vi "Write lasDiodeData.vi"(8 "error in":errorcluster, 10 "lasDiodeData":waveform(i16), 11 "PAS Cell Data in":refnum<class "PAS Cell Data.lvclass">) -> (0 "error out":errorcluster, 3 "PAS Cell Data out":refnum<class "PAS Cell Data.lvclass">)   [LabVIEW 2018, in "PAS Library.lvlib" / "PAS Cell Data.lvclass"]
doc: "Write the data collected off of the PAS laser diode to the class instance."
uses:
  PAS Cell Data.lvclass
  PAS Cell Data.lvclass/PAS Cell Data.ctl
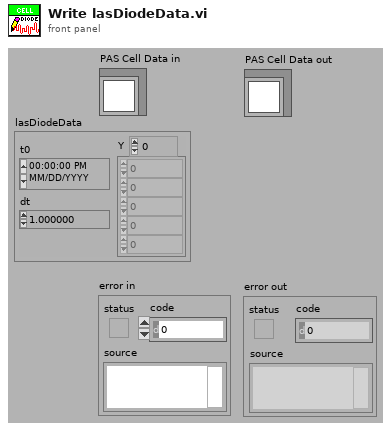
[diagram p1: front panel]
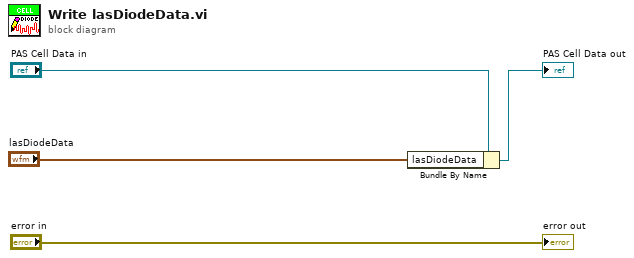
[diagram p0: block diagram]
diagram:
  n1 = Bundle By Name(cluster="PAS Cell Data in", "lasDiodeData"="lasDiodeData") -> (→"PAS Cell Data out":refnum<class "PAS Cell Data.lvclass">)
  "error out" <- "error in"
